vi "Register gRPC Generic Method.vi"(8 "error in (no error)":errorcluster, 11 "Template Server in":refnum<class "Template Server.lvclass">) -> (0 "error out":errorcluster, 3 "Template Server out":refnum<class "Template Server.lvclass">)   [LabVIEW 2019, in "Template Server.lvlib" / "Template Server.lvclass"]
doc: "Registers the generic event if enabled during server initialization.\n\nEnable the generic event if you would like to use a single event for capturing all messages. This would be useful if you are planning to implement your own dispatcher logic. Kindly note that enabling the generic event would not generate the individual events."
uses:
  Template Server.lvclass
  <vilib>/gRPC/LabVIEW gRPC Library/gprc-lvsupport-release.lvlib
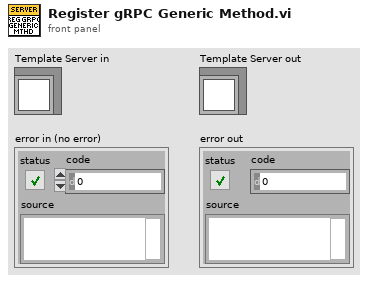
[diagram p1: front panel]
types:
  T1 = typedef "gprc-lvsupport-release.lvlib/grpcId.ctl" = u64
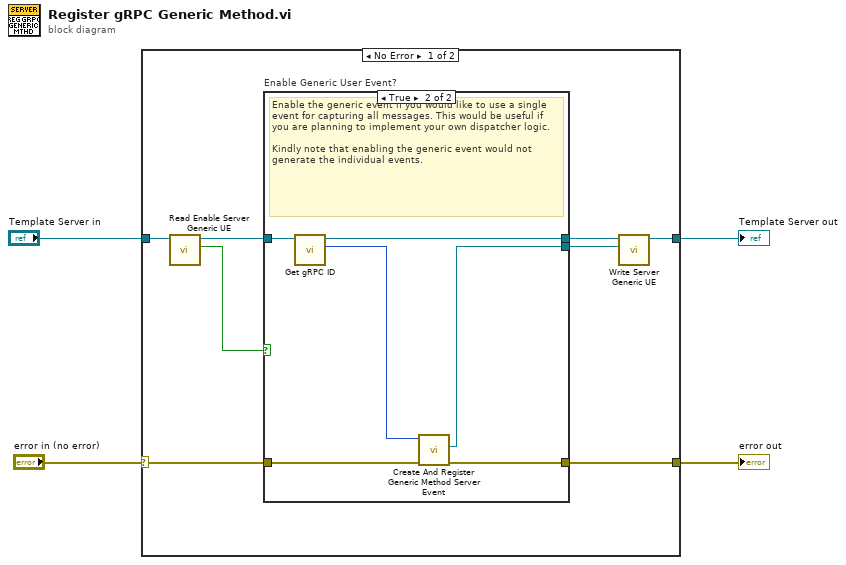
[diagram p0: block diagram]
diagram:
  n1 = case shown="No Error" "error in (no error)" {
    selector: "error in (no error)" -> [w12 w21]
    tunnel: "Template Server in" -> [w9 w22]
    tunnel: [w11 w21] -> w3
    tunnel: [w10 w22] -> w2
    frame No Error {
      n2 = call "Read Enable Server Generic UE.vi"("Template Server in"=w9) -> ("Enable Server Generic UE"=w5:bool, "Template Server out"=w8:refnum<class "Template Server.lvclass">)  [unwired: 9 in]
      n3 = case "Enable Generic User Event?" shown="True" w5 {
        tunnel: w12 -> [w13 w20]
        tunnel: [w13 w19] -> w11
        tunnel: w8 -> [w14 w18]
        tunnel: [w14 w17] -> w7
        tunnel: [_ w15] -> w6
        frame False {
        }
        frame True {
          # "Enable the generic event if you would like to use a single event for capturing all messages. This would be useful if you are planning to implement your own dispatcher logic. \n\nKindly note that enabling the generic event would not generate the individual events."
          n4 = call "Get gRPC ID.vi"("OOP Server in"=w18) -> ("gRPC ID"=w16:T1, "OOP Server out"=w17:refnum<class "Template Server.lvclass">)  [unwired: 9 in]
          n5 = call <vilib>:"Create And Register Generic Method Server Event.vi"("error in (no error)"=w20, "gRPCid server in"=w16) -> ("error out"=w19:errorcluster, "Generic Method Event"=w15:refnum<user-event>)  [unwired: 7 in, 1 out]
        }
      }
      n6 = call "Write Server Generic UE.vi"("Server Generic UE"=w6, "Template Server in"=w7) -> ("Template Server out"=w10:refnum<class "Template Server.lvclass">)  [unwired: 9 in]
    }
    frame Error {
    }
  }
  "error out" <- w3
  "Template Server out" <- w2
